vi "Initialize Actor.vi"(7 "Host Name":string, 8 "error in (no error)":errorcluster, 9 "Actor Name":string, 10 "Message Broker Interface":refnum<class "Message Broker Interface.lvclass">, 11 "Mediated Asynchronous Actor in":refnum<class "Mediated Asynchronous Actor.lvclass">) -> (0 "error out":errorcluster, 3 "Mediated Asynchronous Actor out":refnum<class "Mediated Asynchronous Actor.lvclass">)   [LabVIEW 2016, in "Stream Mediator.lvlib" / "Mediated Asynchronous Actor.lvclass"]
doc: "--\nCopyright © 2017 Composed SystemsI All rights reserved.\n\nAuthor: Jon McBee <jon.mcbee@composed.io>\n\nThis library is provided \"AS IS\" ,WITHOUT WARRANTIES OR\nCONDITIONS OF ANY KIND, either express or implied.\n\nComposed Systems -- composed.io\n\nStream 0.0.1.1\nJon McBee - Composed Systems\nCopyright (c) 2017, Composed Systems"
uses:
  <userlib>/Composed Systems/Stream/Mediator/Classes/Mediated Asynchronous Actor/Mediated Asynchronous Actor.lvclass
  C:/Program Files (x86)/National Instruments/LabVIEW 2016/user.lib/Composed Systems/Stream/Actor/Actor Class/Ancestral Actor.lvclass
  <userlib>/Composed Systems/Stream/Mediator/Classes/Message Broker Interface/Message Broker Interface.lvclass
  <userlib>/Composed Systems/Stream/Mediator/Classes/Mediated Asynchronous Actor/Mediated Asynchronous Actor.lvclass/Mediated Asynchronous Actor.ctl
  <userlib>/Composed Systems/Stream/Actor/Actor Class/Ancestral Actor.lvclass/Ancestral Actor.ctl
  <userlib>/Composed Systems/Stream/Mediator/Classes/Message Transport Queue/Message Transport Queue.lvclass
  C:/Program Files (x86)/National Instruments/LabVIEW 2016/user.lib/Composed Systems/Stream/Mediator/Classes/Message Transport Interface/Message Transport Interface.lvclass
  <userlib>/Composed Systems/Stream/Mediator/Classes/Mediated Actor/Mediated Actor.lvclass
  <userlib>/Composed Systems/Stream/Actor/Actor Class/Ancestral Actor.lvclass
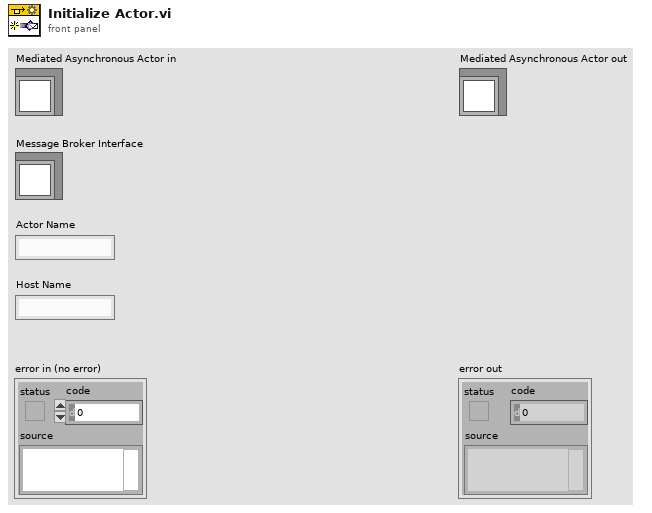
[diagram p1: front panel]
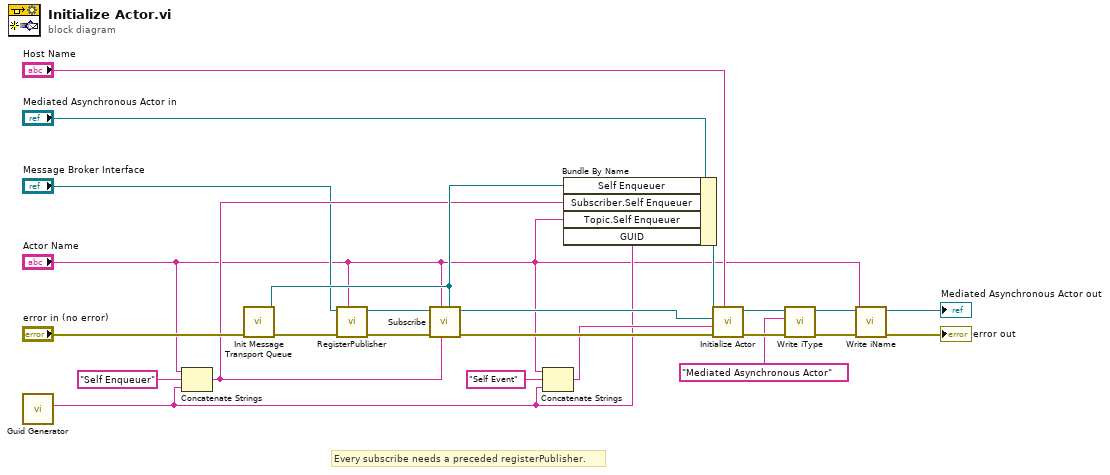
[diagram p0: block diagram]
diagram:
  # "Every subscribe needs a preceded registerPublisher."
  n1 = call <vilib>:"Guid Generator.vi"() -> ("GUID"=w5:string)  [unwired: 10 in, 1 out]
  n2 = Concatenate Strings("Actor Name", "Self Enqueuer" ("string"), w5) -> (w13:string)
  n3 = call <userlib>:"Init Message Transport Queue.vi"("error in (no error)"="error in (no error)") -> ("error out"=w21:errorcluster, "Message Transport Queue out"=w15:refnum<class "Message Transport Queue.lvclass">)  [unwired: 9 in]
  n4 = call-dynamic "RegisterPublisher.vi"("Topic Name"="Actor Name", "error in (no error)"=w21, "Message Broker Interface in"="Message Broker Interface") -> ("error out"=w4:errorcluster, "Message Broker Interface out"=w2:refnum<class "Message Broker Interface.lvclass">)  [unwired: 4 in, 3 out]
  n5 = call-dynamic "Subscribe.vi"("Message Transport Interface"=w15, "Subscriber Name"=w13, "Topic Name"="Actor Name", "error in (no error)"=w4, "Message Broker Interface in"=w2) -> ("error out"=w19:errorcluster, "Message Broker Interface out"=w18:refnum<class "Message Broker Interface.lvclass">)  [unwired: 4 in, 1 out]
  n6 = Concatenate Strings("Actor Name", "Self Event" ("string"), w5) -> (w14:string)
  n7 = Bundle By Name(cluster="Mediated Asynchronous Actor in", "Self Enqueuer"=w15, "Subscriber.Self Enqueuer"=w13, "Topic.Self Enqueuer"="Actor Name", "GUID"=w5) -> (w16:refnum<class "Mediated Asynchronous Actor.lvclass">)
  n8 = call-parent "Initialize Actor.vi"("Host Name"="Host Name", "error in (no error)"=w19, "Actor Name"=w14, "Message Broker Interface"=w18, "Mediated Actor in"=w16) -> ("error out"=w12:errorcluster, "Mediated Actor out"=w11:refnum<class "Mediated Asynchronous Actor.lvclass">)  [unwired: 5 in]
  n9 = call <userlib>:"Write iType.vi"("error in (no error)"=w12, "iType"="Mediated Asynchronous Actor", "Ancestral Actor in"=w11) -> ("error out"=w10:errorcluster, "Ancestral Actor out"=w8:refnum<class "Mediated Asynchronous Actor.lvclass">)  [unwired: 7 in]
  n10 = call <userlib>:"Write iName.vi"("error in (no error)"=w10, "iName"="Actor Name", "Ancestral Actor in"=w8) -> ("error out"=→"error out":errorcluster, "Ancestral Actor out"=→"Mediated Asynchronous Actor out":refnum<class "Mediated Asynchronous Actor.lvclass">)  [unwired: 7 in]
